vi "FTW-Connector-LaunchActor.vi"(0 "FTW Actor Connector Type":refnum<class "FTW-ActorConnector.lvclass">, 7 "Configuration":string, 11 "error in":errorcluster) -> (4 "FTW Actor Connector":refnum<class "FTW-ActorConnector.lvclass">, 15 "error out":errorcluster)   [LabVIEW 2015, in "FTW-ActorConnector.lvclass"]
uses:
  FTW-ActorConnector.lvclass
  Instance/FTW-ActorInstance.lvclass
  Instance/FTW-Actor-AsyncLaunch.vi
panel:
  # "Inputs"
  # "Outputs"
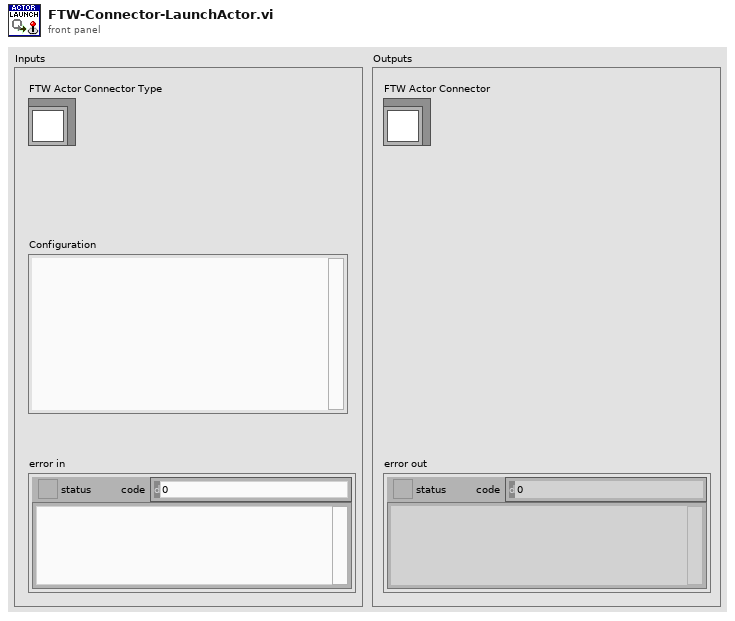
[diagram p1: front panel]
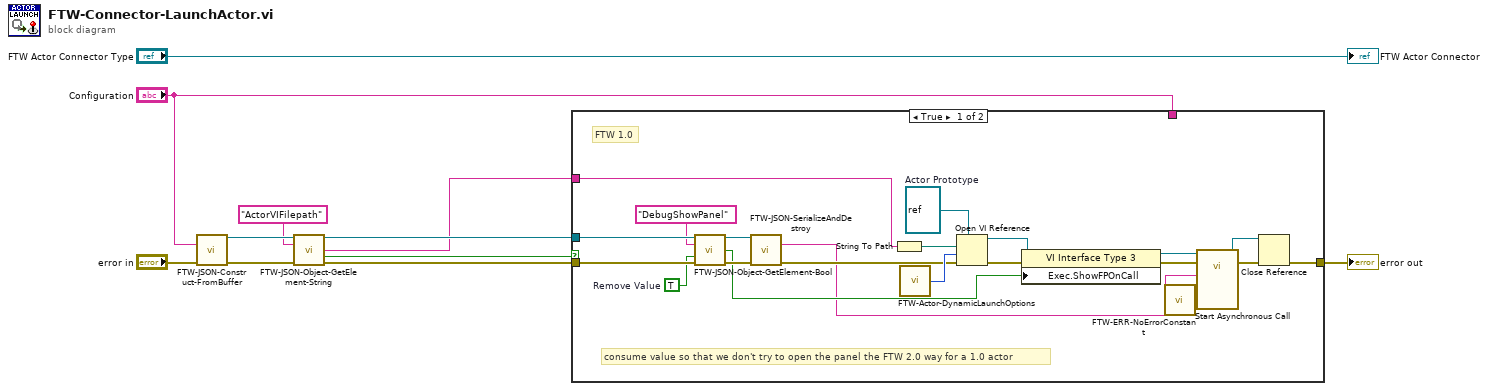
[diagram p0: block diagram]
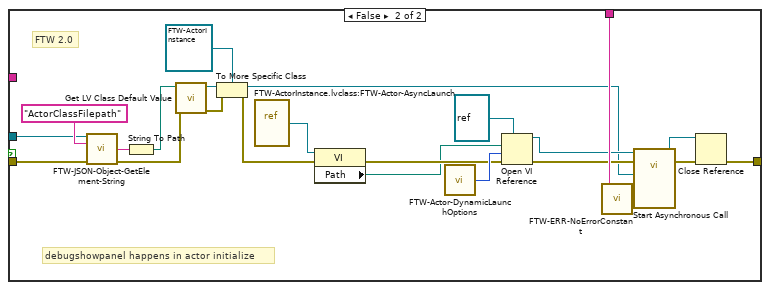
[diagram p2: hidden frame]
diagram:
  n1 = call "FTW-JSON-Construct-FromBuffer.vi"("JSON String (UTF-8)"="Configuration", "error in"="error in") -> ("JSON"=w5:refnum<class "FTW-Container.lvclass">, "error out"=w8:errorcluster)  [unwired: 12 in]
  n2 = call "FTW-JSON-Object-GetElement-String.vi"("JSON"=w5, "Key"="ActorVIFilepath", "error in"=w8) -> ("JSON out"=w2:refnum<class "FTW-Container.lvclass">, "Value"=w1:string, "Found"=w3:bool, "error out"=w6:errorcluster)  [unwired: 8 in, 1 out]
  n3 = case shown="True" w3 {
    tunnel: [w32 w54] -> w11
    tunnel: "Configuration" -> [_ w53]
    tunnel: w6 -> [w23 w41]
    tunnel: w2 -> [w19 w34]
    tunnel: w1 -> [w15 _]
    frame True {
      w17 = TRUE  # Remove Value
      w31 = refnum<vi> refnum  # Actor Prototype
      # "consume value so that we don't try to open the panel the FTW 2.0 way for a 1.0 actor"
      # "FTW 1.0"
      n4 = call "FTW-JSON-Object-GetElement-Bool.vi"("JSON"=w19, "Key"="DebugShowPanel", "Remove Value"=w17, "error in"=w23) -> ("JSON out"=w13:refnum<class "FTW-Container.lvclass">, "Value"=w16:bool, "error out"=w20:errorcluster)  [unwired: 8 in, 1 out]
      n5 = call "FTW-JSON-SerializeAndDestroy.vi"("JSON"=w13, "error in"=w20) -> ("JSON String (UTF-8)"=w12:string, "error out"=w14:errorcluster)  [unwired: 12 in]
      n6 = String To Path(string=w15) -> (path=w21:path)
      n7 = call "FTW-Actor-DynamicLaunchOptions.vi"() -> ("Open VI Ref Options"=w30:i32)
      n8 = Open VI Reference(type specifier VI Refnum (for type only)=w31, vi path=w21, options=w30, error in (no error)=w14) -> (vi reference=w24:refnum<vi>, error out=w22:errorcluster)  [unwired: 2 in]
      n9 = property class="VI Interface Type 3"(reference=w24, error in=w22, "Exec.ShowFPOnCall"=w16) -> (reference out=w26:refnum<vi>, error out=w25:errorcluster)
      n10 = call "FTW-ERR-NoErrorConstant.vi"() -> ("no error"=w29:errorcluster)
      n11 = call-by-ref "Start Asynchronous Call"(reference=w26, error in=w25, "Configuration"=w12, "ErrorIn"=w29) -> (reference out=w28:refnum<vi>, error out=w27:errorcluster)  [unwired: 13 in, 1 out]
      n12 = Close Reference(reference=w28, error in (no error)=w27) -> (error out=w32:errorcluster)
    }
    frame False {
      # "debugshowpanel happens in actor initialize"
      # "FTW 2.0"
      n13 = call "FTW-JSON-Object-GetElement-String.vi"("JSON"=w34, "Key"="ActorClassFilepath") -> ("Value"=w33:string)  [unwired: 9 in, 4 out]
      n14 = String To Path(string=w33) -> (path=w46:path)
      n15 = call <vilib>:"Get LV Class Default Value.vi"("error in (no error)"=w41, "class path"=w46) -> ("error out"=w43:errorcluster, "object"=w45:refnum<class>)  [unwired: 8 in]
      n16 = To More Specific Class(target class=refnum<class "FTW-ActorInstance.lvclass"> refnum ("FTW Actor Instance"), reference=w45, error in=w43) -> (specific class reference=w42:refnum<class "FTW-ActorInstance.lvclass">, error out=w40:errorcluster)
      n17 = vi-ref "FTW-ActorInstance.lvclass:FTW-Actor-AsyncLaunch.vi"() -> (w38:refnum<vi>)
      n18 = property class="VI"(reference=w38, error in=w40) -> (error out=w39:errorcluster, "Path"=w37:path)  [unwired: 1 out]
      n19 = call "FTW-Actor-DynamicLaunchOptions.vi"() -> ("Open VI Ref Options"=w52:i32)
      n20 = Open VI Reference(type specifier VI Refnum (for type only)=refnum<vi> refnum, vi path=w37, options=w52, error in (no error)=w39) -> (vi reference=w48:refnum<vi>, error out=w47:errorcluster)  [unwired: 2 in]
      n21 = call "FTW-ERR-NoErrorConstant.vi"() -> ("no error"=w51:errorcluster)
      n22 = call-by-ref "Start Asynchronous Call"(reference=w48, error in=w47, "FTW Actor Instance Type"=w42, "Actor Instance Configuration"=w53, "error in"=w51) -> (reference out=w50:refnum<vi>, error out=w49:errorcluster)  [unwired: 12 in, 1 out]
      n23 = Close Reference(reference=w50, error in (no error)=w49) -> (error out=w54:errorcluster)
    }
  }
  "error out" <- w11
  "FTW Actor Connector" <- "FTW Actor Connector Type"
